vi "eTdsBLE_Debug.vi"() -> ()   [LabVIEW 2013]
panel:
  in  "stop":bool
  out "error out":errorcluster
  out "BleDataArray":u8[](array[numeric])
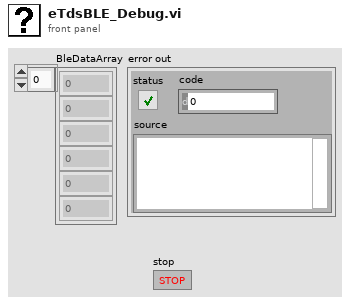
[diagram p1: front panel]
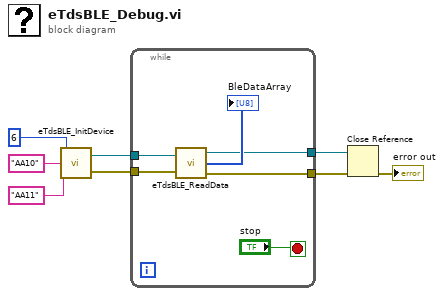
[diagram p0: block diagram]
diagram:
  n1 = call "eTdsBLE_InitDevice.vi"("characteristicUUID"="AA11", "serviceUUID"="AA10", "NumEltDataArray"=6) -> ("error out"=w4:errorcluster, "eTdsDevice Reference"=w5:refnum<k24>)
  n2 = while {
    tunnel: w5 -> [w14]
    tunnel: w4 -> [w13]
    tunnel: [w11] -> w3
    tunnel: [w10] -> w2
    stop <- "stop" stop-if-true
    n3 = call "eTdsBLE_ReadData.vi"("eTDS Reference"=w14, "error in"=w13) -> ("eTDS Ref Out"=w11:refnum<k24>, "BleDataArray"=→"BleDataArray":u8[], "error out"=w10:errorcluster)
  }
  n4 = Close Reference(reference=w3, error in (no error)=w2) -> (error out=→"error out":errorcluster)
